vi "MODBUS  SLAVE.vi"() -> (3 "values to write":u16[](array[numeric]) caption="待写入值")   [LabVIEW 2016]
uses:
  <vilib>/Modbus/subvis/Data and Functions/Device Data Model/Device Data Model.lvclass
  <vilib>/Modbus/slave/Create Slave Instance (TCP).vi
  <vilib>/Modbus/slave/Modbus Slave.lvclass
  API/CodCr/CodCr.lvlib
panel:
  out "运行周期":u16[](array[numeric])
  in  "write operation starting address":u16=100 caption="写操作起始地址"
  out "单仪器启动命令":u16[](array[numeric])
  out "系统启动命令":u16[](array[numeric])
  in  "停止":bool
  out "register values":u16[](array[numeric]) caption="寄存器值"
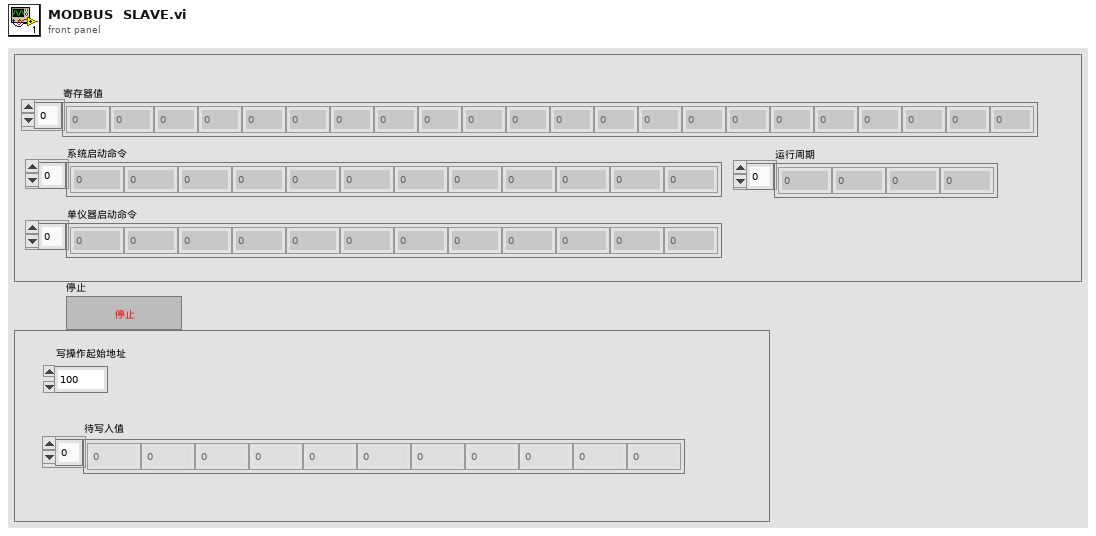
[diagram p1: front panel]
types:
  T1 = cluster{"测量模式":enum16{"水样测量", "标样核查", "零点核查", "跨度核查", "空白测试", "加标回收", "平行样", "校零", "校标"}}
  T2 = cluster{"站号":u16, "量程切换":enum32{"H", "L", "AUTO"}, "控制命令":enum16{"启动测量", "标样核查", "零点核查", "跨度核查", "空白测试", "平行样测试", "加标回收", "空白校准", "标样校准", "初始化（清洗）", "停止测试", "仪器重启", "校时", "模式设置", "测量间隔设置"}, "模式设置":enum16{"待机", "连续模式", "周期模式", "定点模式", "受控模式", "手动模式"}, "测量间隔":u16}
  T3 = cluster{"测量模式":enum16{"水样测量", "标样核查", "零点核查", "跨度核查", "加标回收", "平行样", "校零", "校标"}}
  T4 = cluster{"系统时间":timestamp, "工作状态":enum16{"空闲", "水样测试", "标样核查", "零点核查", "跨度核查", "空白测试", "平行样测试", "加标回收", "空白校准", "标样校准", "初始化（清洗）"}, "测量模式":enum16{"待机", "连续模式", "周期模式", "定点模式", "受控模式", "手动模式"}, "告警代码":enum16{"无告警", "缺试剂告警", "缺水样告警", "缺蒸馏水告警", "缺标液告警", "仪表漏液告警", "标定异常告警", "超量程告警", "加热异常", "低试剂预警", "超上限告警", "超下限告警", "仪表内部其他异常", "滴定异常告警", "电极异常告警", "量程切换告警", "参数设置告警", "PH电极电位异常", "电导率电极异常", "浊度光度异常", "溶解氧电极异常", "溶解氧光强异常", "温度异常告警", "PH异常告警", "溶解氧异常告警", "电导率异常告警", "浊度异常告警", "叶绿素异常告警", "藻密度异常告警", "蓝绿藻异常告警", "ORP异常告警", "氨氮异常告警", "清洁刷异常告警", "SD卡异常告警", "蓝牙异常告警", "Wifi异常告警", "流程异常告警"}, "故障代码":enum16{"无故障", "电机故障", "温度故障", "通讯故障", "滴定故障"}, "日志代码":u16, "软件版本":u16, "F0":sgl, "F1":sgl, "F2":sgl, "F3":sgl, "T":sgl, "H":sgl, "id":u16, "flowid":u16, "量程":u16, "总磷控温温度1":sgl, "营养盐控温温度2":sgl, "ADC":sgl}
  T5 = enum16{"空闲", "水样测试", "标样核查", "零点核查", "跨度核查", "空白测试", "平行样测试", "加标回收", "空白校准", "标样校准", "初始化（清洗）"}
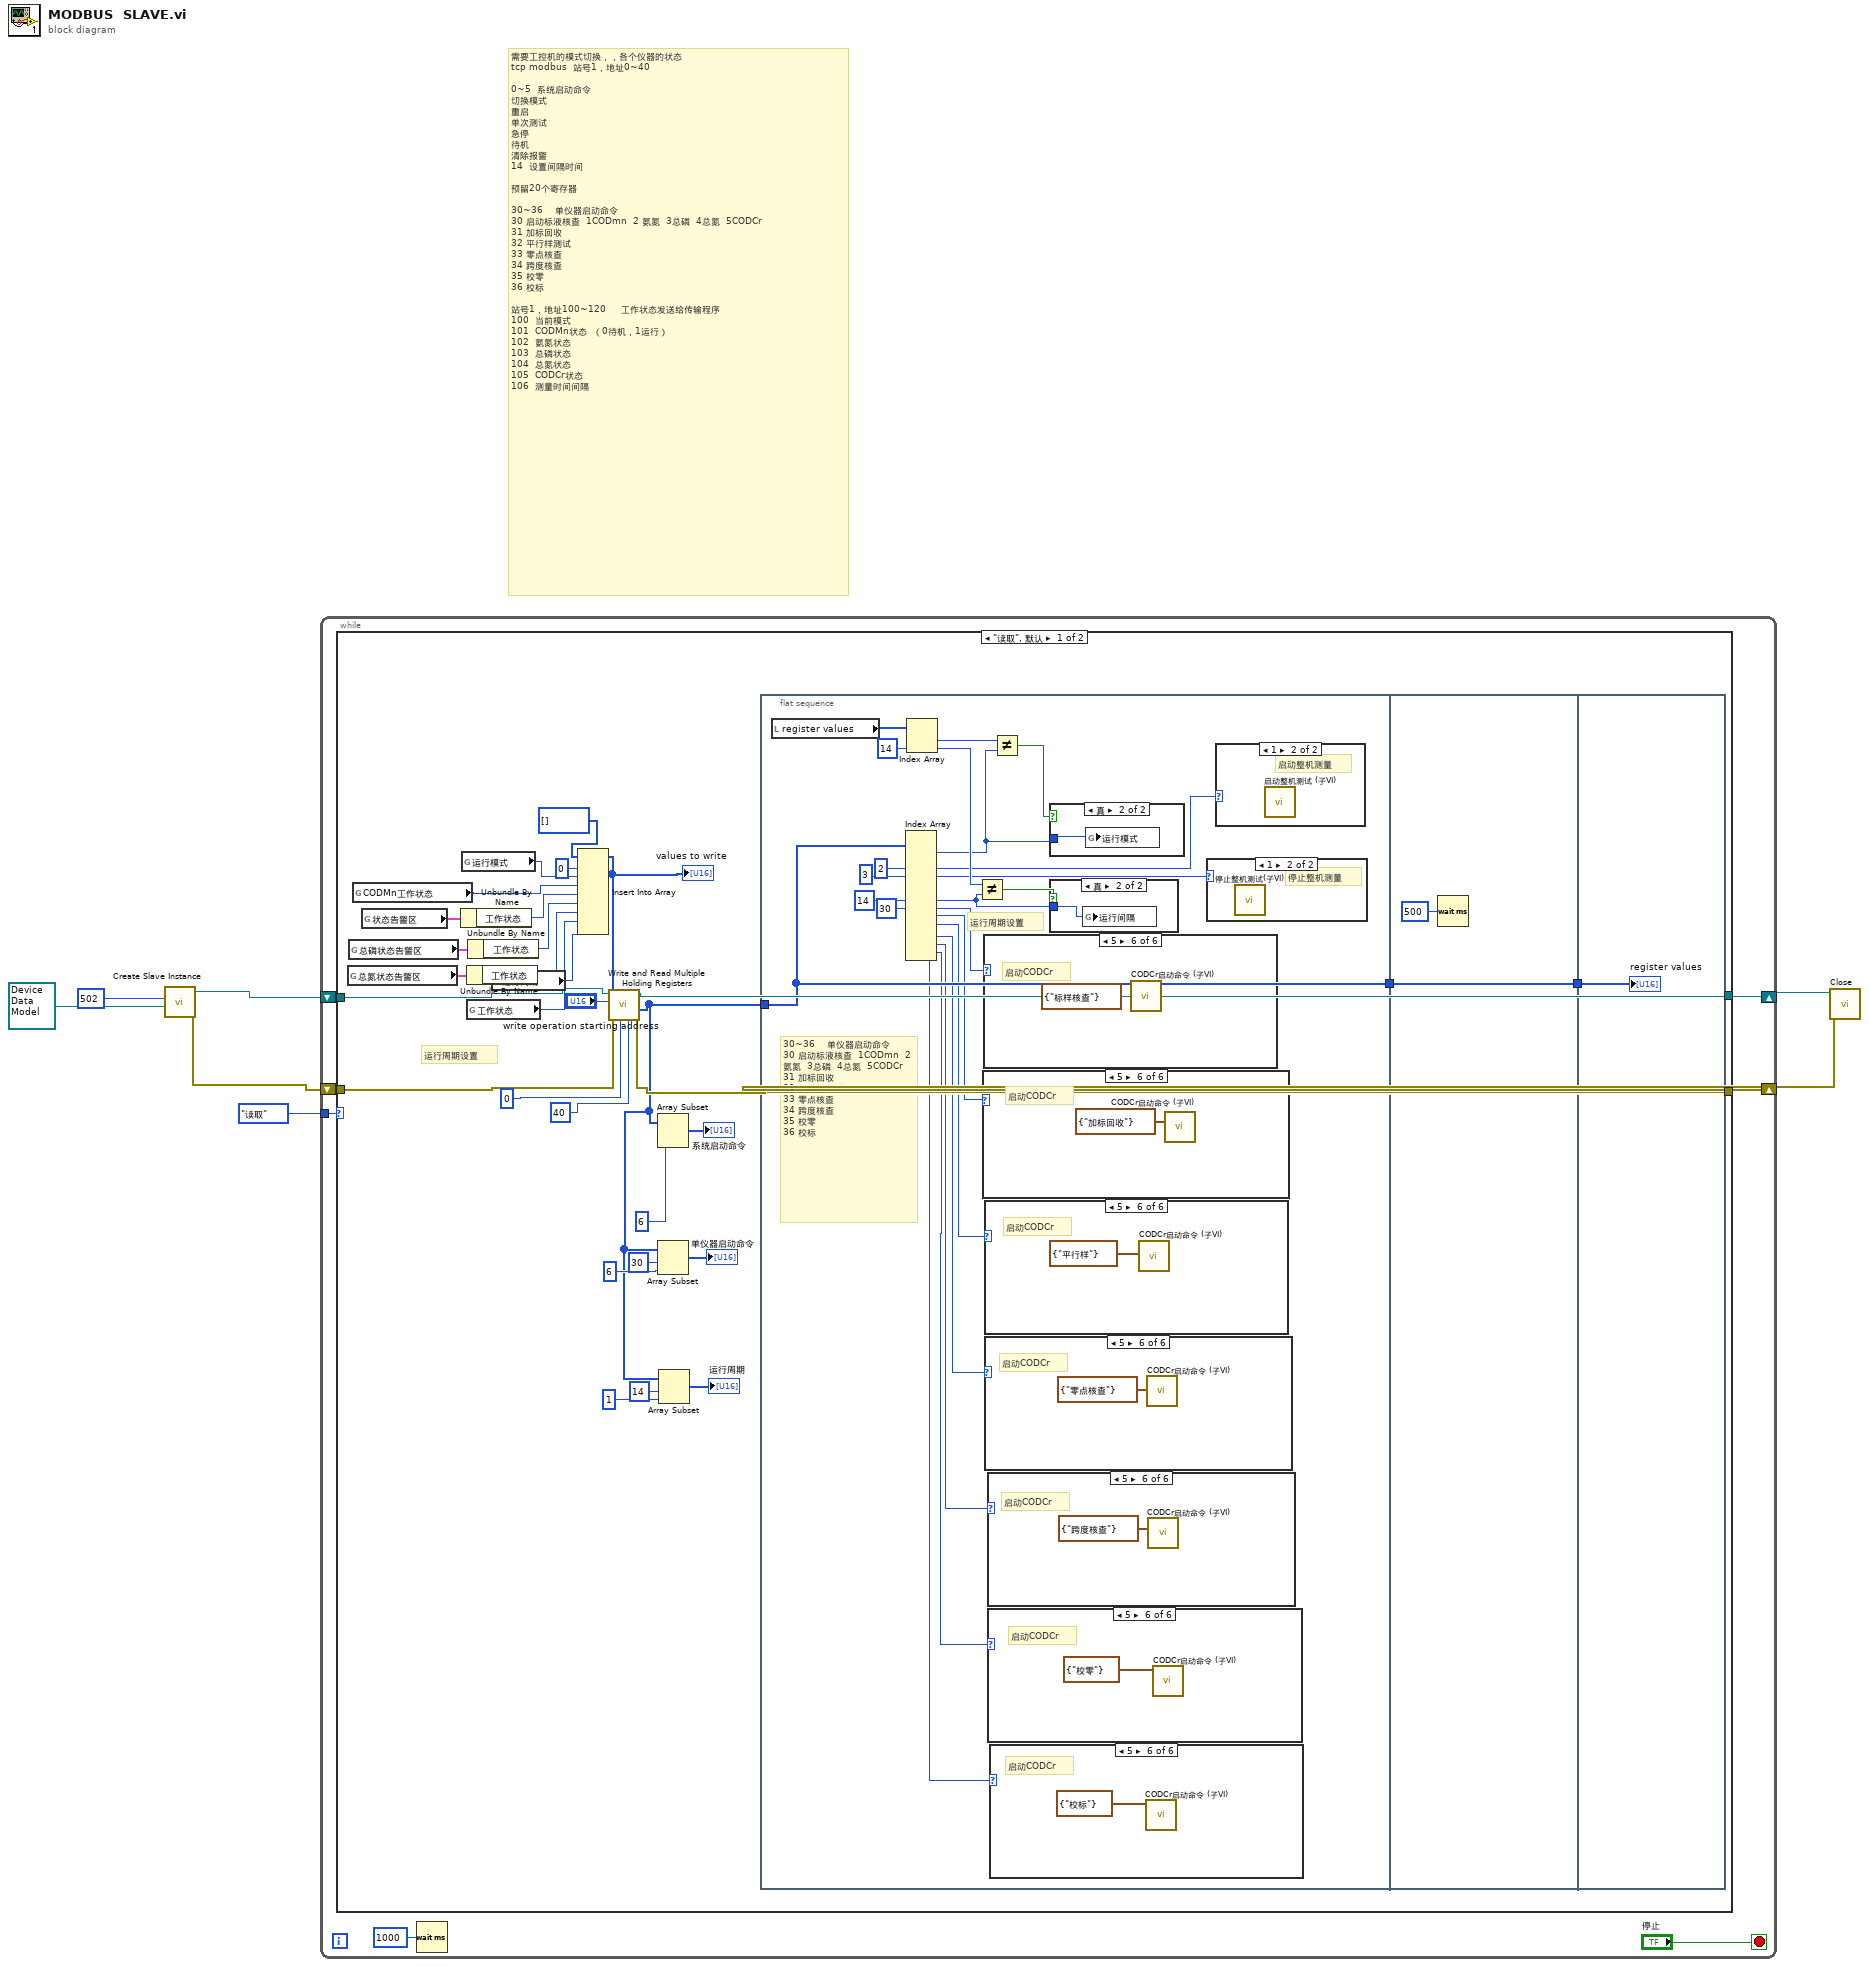
[diagram p0: block diagram]
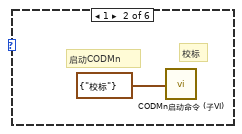
[diagram p3: hidden frame]
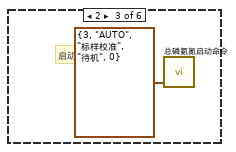
[diagram p4: hidden frame]
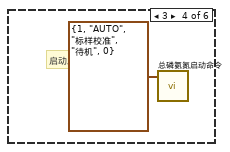
[diagram p5: hidden frame]
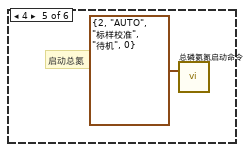
[diagram p6: hidden frame]
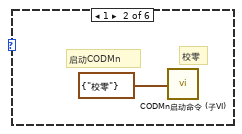
[diagram p8: hidden frame]
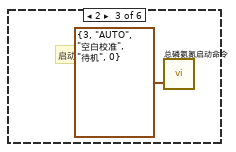
[diagram p9: hidden frame]
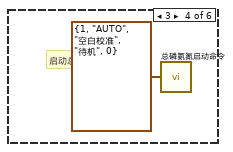
[diagram p10: hidden frame]
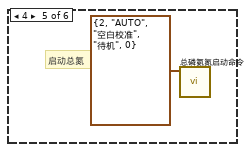
[diagram p11: hidden frame]
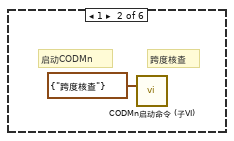
[diagram p13: hidden frame]
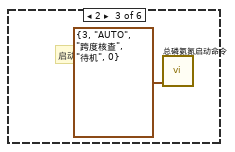
[diagram p14: hidden frame]
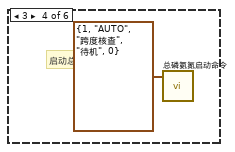
[diagram p15: hidden frame]
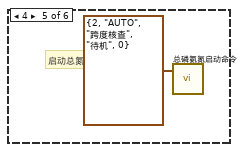
[diagram p16: hidden frame]
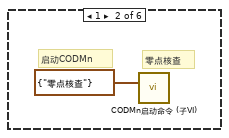
[diagram p18: hidden frame]
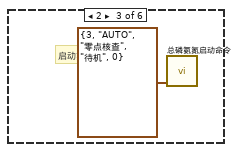
[diagram p19: hidden frame]
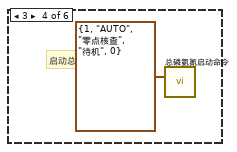
[diagram p20: hidden frame]
diagram:
  # "需要工控机的模式切换，，各个仪器的状态\ntcp modbus  站号1，地址0~40\n\n0~5  系统启动命令\n切换模式\n重启\n单次测试\n急停\n待机\n清除报警\n14  设置间隔时间\n\n预留20个寄存器\n\n30~36    单仪器启动命令\n30 启动标液核查  1CODmn  2 氨氮  3总磷  4总氮  5CODCr\n31 加标回收\n32 平行样测试\n33 零点核查\n34 跨度核查\n35 校零\n36 校标\n\n站号1，地址100~120     工作状态发送给传输程序\n100  当前模式\n101  CODMn状态  （0待机，1运行）\n102  氨氮状态\n103  总磷状态\n104  总氮状态\n105  CODCr状态\n106  测量时间间隔"
  n1 = call-poly <vilib>:"Create Slave Instance.vi"("device data model"=refnum<class "Device Data Model.lvclass"> refnum, "port (502)"=u16 502) -> ("error out"=w5:errorcluster, "TCP slave instance"=w4:refnum<class "Modbus Slave.lvclass">)  [unwired: 8 in]
  n2 = while {
    shift-right: [w12] -> w3
    shift-left: w4 -> [w14]
    shift-right: [w8] -> w2
    shift-left: w5 -> [w13]
    tunnel: enum16{"读取", "写入"}."读取" -> [w9]
    stop <- "停止" stop-if-true
    n3 = case shown="\"读取\", 默认" w9 {
      tunnel: w14 -> [w41 w109]
      tunnel: w13 -> [w40 w108]
      tunnel: [w36 w109] -> w12
      tunnel: [w37 w108] -> w8
      frame "读取", Default {
        # "运行周期设置"
        n4 = global read "VAR总磷氨氮全局变量.vi" "总氮状态告警区"() -> (w19:T4)
        n5 = global read "VAR总磷氨氮全局变量.vi" "总磷状态告警区"() -> (w21:T4)
        n6 = global read "COD测量模式全局.vi" "CODMn工作状态"() -> (w17:T5)
        n7 = global read "VAR总磷氨氮全局变量.vi" "状态告警区"() -> (w23:T4)
        n8 = Unbundle By Name(w23) -> ("工作状态"=w22:T5)
        n9 = global read "系统变量.vi" "运行模式"() -> (w33:enum16{"维护模式", "常规模式", "应急模式", "质控模式"})
        n10 = Unbundle By Name(w19) -> ("工作状态"=w18:T5)
        n11 = global read "CODcr全局变量.vi" "工作状态"() -> (w16:T5)
        n12 = Unbundle By Name(w21) -> ("工作状态"=w20:T5)
        n13 = global read "系统变量.vi" "运行间隔"() -> (w15:i16)
        n14 = Insert Into Array(array=u16[] [] ("values to write"), index=0 ("索引"), new element #1=w33, new element #2=w17, new element #3=w22, new element #4=w20, new element #5=w18, new element #6=w16, new element #7=w15) -> (w31:u16[])
        "values to write" <- w31
        n15 = call-dynamic "Write and Read Multiple Holding Registers.vi"("read count"=u16 40 ("number of holding registers"), "read operation starting address"=u16 0 ("starting address"), "error in (no error)"=w40, "values to write"=w31, "write operation starting address"="write operation starting address", "Modbus slave in"=w41) -> ("error out"=w37:errorcluster, "values read"=w26:u16[], "Modbus slave out"=w36:refnum<class "Modbus Slave.lvclass">)  [unwired: 3 in]
        n16 = Array Subset(array=w26, length=6 ("长度")) -> (→"系统启动命令":u16[])  [unwired: 1 in]
        n17 = Array Subset(array=w26, index=30 ("索引"), length=6 ("长度")) -> (→"单仪器启动命令":u16[])
        n18 = Array Subset(array=w26, index=14 ("索引"), length=1 ("长度")) -> (→"运行周期":u16[])
        n19 = flat-sequence {
          tunnel: w26 -> [w67]
          tunnel: [w67] -> w25
          tunnel: w25 -> [w105]
          tunnel: [w105] -> w24
          tunnel: w24 -> [w107]
          frame #0 {
            # "运行周期设置"
            # "30~36    单仪器启动命令\n30 启动标液核查  1CODmn  2 氨氮  3总磷  4总氮  5CODCr\n31 加标回收\n32 平行样测试\n33 零点核查\n34 跨度核查\n35 校零\n36 校标"
            n20 = local read "register values"() -> (w66:u16[])
            n21 = Index Array(array=w67, index #3=2 ("索引"), index #4=3 ("索引"), index #7=14 ("索引"), index #8=30 ("索引")) -> (element #1=w54:u16, element #3=w55:u16, element #4=w56:u16, element #7=w57:u16, element #8=w52:u16, element #9=w51:u16, element #10=w50:u16, element #11=w49:u16, element #12=w48:u16, element #13=w47:u16, element #14=w46:u16)  [unwired: 10 in, 3 out]
            n22 = Index Array(array=w66, index #2=14 ("索引")) -> (element #1=w65:u16, element #2=w62:u16)  [unwired: 1 in]
            n23 = Not Equal?(x=w62, y=w57) -> (x != y?=w61:bool)
            n24 = case shown="5" w51 {
              frame 0, Default {
              }
              frame 1 {
                # "加标回收"
                # "启动CODMn"
                n25 = call "CODMn启动命令 (子VI).vi"("启动测量模式"=T1 {"测量模式"=enum."加标回收"}) -> ()  [unwired: 11 in]
              }
              frame 2 {
                # "启动氨氮"
                n26 = call "总磷氨氮启动命令.vi"("参数"=T2 {"站号"=3, "量程切换"=enum."AUTO", "控制命令"=enum."加标回收", "模式设置"=enum."待机", "测量间隔"=0}) -> ()  [unwired: 10 in, 1 out]
              }
              frame 3 {
                # "启动总磷"
                n27 = call "总磷氨氮启动命令.vi"("参数"=T2 {"站号"=1, "量程切换"=enum."AUTO", "控制命令"=enum."加标回收", "模式设置"=enum."待机", "测量间隔"=0}) -> ()  [unwired: 10 in, 1 out]
              }
              frame 4 {
                # "启动总氮"
                n28 = call "总磷氨氮启动命令.vi"("参数"=T2 {"站号"=2, "量程切换"=enum."AUTO", "控制命令"=enum."加标回收", "模式设置"=enum."待机", "测量间隔"=0}) -> ()  [unwired: 10 in, 1 out]
              }
              frame 5 {
                # "启动CODCr"
                n29 = call "CODCr启动命令 (子VI).vi"("启动测量模式"=T3 {"测量模式"=enum."加标回收"}) -> ()  [unwired: 11 in]
              }
            }
            n30 = case shown="5" w52 {
              frame 0, Default {
              }
              frame 1 {
                # "启动标液核查"
                # "启动CODMn"
                n31 = call "CODMn启动命令 (子VI).vi"("启动测量模式"=T1 {"测量模式"=enum."标样核查"}) -> ()  [unwired: 11 in]
              }
              frame 2 {
                # "启动氨氮"
                n32 = call "总磷氨氮启动命令.vi"("参数"=T2 {"站号"=3, "量程切换"=enum."AUTO", "控制命令"=enum."标样核查", "模式设置"=enum."待机", "测量间隔"=0}) -> ()  [unwired: 10 in, 1 out]
              }
              frame 3 {
                # "启动总磷"
                n33 = call "总磷氨氮启动命令.vi"("参数"=T2 {"站号"=1, "量程切换"=enum."AUTO", "控制命令"=enum."标样核查", "模式设置"=enum."待机", "测量间隔"=0}) -> ()  [unwired: 10 in, 1 out]
              }
              frame 4 {
                # "启动总氮"
                n34 = call "总磷氨氮启动命令.vi"("参数"=T2 {"站号"=2, "量程切换"=enum."AUTO", "控制命令"=enum."标样核查", "模式设置"=enum."待机", "测量间隔"=0}) -> ()  [unwired: 10 in, 1 out]
              }
              frame 5 {
                # "启动CODCr"
                n35 = call "CODCr启动命令 (子VI).vi"("启动测量模式"=T3 {"测量模式"=enum."标样核查"}) -> ()  [unwired: 11 in]
              }
            }
            n36 = case shown="5" w50 {
              frame 0, Default {
              }
              frame 1 {
                # "平行样测试"
                # "启动CODMn"
                n37 = call "CODMn启动命令 (子VI).vi"("启动测量模式"=T1 {"测量模式"=enum."平行样"}) -> ()  [unwired: 11 in]
              }
              frame 2 {
                # "启动氨氮"
                n38 = call "总磷氨氮启动命令.vi"("参数"=T2 {"站号"=3, "量程切换"=enum."AUTO", "控制命令"=enum."平行样测试", "模式设置"=enum."待机", "测量间隔"=0}) -> ()  [unwired: 10 in, 1 out]
              }
              frame 3 {
                # "启动总磷"
                n39 = call "总磷氨氮启动命令.vi"("参数"=T2 {"站号"=1, "量程切换"=enum."AUTO", "控制命令"=enum."平行样测试", "模式设置"=enum."待机", "测量间隔"=0}) -> ()  [unwired: 10 in, 1 out]
              }
              frame 4 {
                # "启动总氮"
                n40 = call "总磷氨氮启动命令.vi"("参数"=T2 {"站号"=2, "量程切换"=enum."AUTO", "控制命令"=enum."平行样测试", "模式设置"=enum."待机", "测量间隔"=0}) -> ()  [unwired: 10 in, 1 out]
              }
              frame 5 {
                # "启动CODCr"
                n41 = call "CODCr启动命令 (子VI).vi"("启动测量模式"=T3 {"测量模式"=enum."平行样"}) -> ()  [unwired: 11 in]
              }
            }
            n42 = case shown="5" w49 {
              frame 0, Default {
              }
              frame 1 {
                # "零点核查"
                # "启动CODMn"
                n43 = call "CODMn启动命令 (子VI).vi"("启动测量模式"=T1 {"测量模式"=enum."零点核查"}) -> ()  [unwired: 11 in]
              }
              frame 2 {
                # "启动氨氮"
                n44 = call "总磷氨氮启动命令.vi"("参数"=T2 {"站号"=3, "量程切换"=enum."AUTO", "控制命令"=enum."零点核查", "模式设置"=enum."待机", "测量间隔"=0}) -> ()  [unwired: 10 in, 1 out]
              }
              frame 3 {
                # "启动总磷"
                n45 = call "总磷氨氮启动命令.vi"("参数"=T2 {"站号"=1, "量程切换"=enum."AUTO", "控制命令"=enum."零点核查", "模式设置"=enum."待机", "测量间隔"=0}) -> ()  [unwired: 10 in, 1 out]
              }
              frame 4 {
                # "启动总氮"
                n46 = call "总磷氨氮启动命令.vi"("参数"=T2 {"站号"=2, "量程切换"=enum."AUTO", "控制命令"=enum."零点核查", "模式设置"=enum."待机", "测量间隔"=0}) -> ()  [unwired: 10 in, 1 out]
              }
              frame 5 {
                # "启动CODCr"
                n47 = call "CODCr启动命令 (子VI).vi"("启动测量模式"=T3 {"测量模式"=enum."零点核查"}) -> ()  [unwired: 11 in]
              }
            }
            n48 = case shown="5" w48 {
              frame 0, Default {
              }
              frame 1 {
                # "跨度核查"
                # "启动CODMn"
                n49 = call "CODMn启动命令 (子VI).vi"("启动测量模式"=T1 {"测量模式"=enum."跨度核查"}) -> ()  [unwired: 11 in]
              }
              frame 2 {
                # "启动氨氮"
                n50 = call "总磷氨氮启动命令.vi"("参数"=T2 {"站号"=3, "量程切换"=enum."AUTO", "控制命令"=enum."跨度核查", "模式设置"=enum."待机", "测量间隔"=0}) -> ()  [unwired: 10 in, 1 out]
              }
              frame 3 {
                # "启动总磷"
                n51 = call "总磷氨氮启动命令.vi"("参数"=T2 {"站号"=1, "量程切换"=enum."AUTO", "控制命令"=enum."跨度核查", "模式设置"=enum."待机", "测量间隔"=0}) -> ()  [unwired: 10 in, 1 out]
              }
              frame 4 {
                # "启动总氮"
                n52 = call "总磷氨氮启动命令.vi"("参数"=T2 {"站号"=2, "量程切换"=enum."AUTO", "控制命令"=enum."跨度核查", "模式设置"=enum."待机", "测量间隔"=0}) -> ()  [unwired: 10 in, 1 out]
              }
              frame 5 {
                # "启动CODCr"
                n53 = call "CODCr启动命令 (子VI).vi"("启动测量模式"=T3 {"测量模式"=enum."跨度核查"}) -> ()  [unwired: 11 in]
              }
            }
            n54 = case shown="5" w47 {
              frame 0, Default {
              }
              frame 1 {
                # "校零"
                # "启动CODMn"
                n55 = call "CODMn启动命令 (子VI).vi"("启动测量模式"=T1 {"测量模式"=enum."校零"}) -> ()  [unwired: 11 in]
              }
              frame 2 {
                # "启动氨氮"
                n56 = call "总磷氨氮启动命令.vi"("参数"=T2 {"站号"=3, "量程切换"=enum."AUTO", "控制命令"=enum."空白校准", "模式设置"=enum."待机", "测量间隔"=0}) -> ()  [unwired: 10 in, 1 out]
              }
              frame 3 {
                # "启动总磷"
                n57 = call "总磷氨氮启动命令.vi"("参数"=T2 {"站号"=1, "量程切换"=enum."AUTO", "控制命令"=enum."空白校准", "模式设置"=enum."待机", "测量间隔"=0}) -> ()  [unwired: 10 in, 1 out]
              }
              frame 4 {
                # "启动总氮"
                n58 = call "总磷氨氮启动命令.vi"("参数"=T2 {"站号"=2, "量程切换"=enum."AUTO", "控制命令"=enum."空白校准", "模式设置"=enum."待机", "测量间隔"=0}) -> ()  [unwired: 10 in, 1 out]
              }
              frame 5 {
                # "启动CODCr"
                n59 = call "CODCr启动命令 (子VI).vi"("启动测量模式"=T3 {"测量模式"=enum."校零"}) -> ()  [unwired: 11 in]
              }
            }
            n60 = case shown="5" w46 {
              frame 0, Default {
              }
              frame 1 {
                # "校标"
                # "启动CODMn"
                n61 = call "CODMn启动命令 (子VI).vi"("启动测量模式"=T1 {"测量模式"=enum."校标"}) -> ()  [unwired: 11 in]
              }
              frame 2 {
                # "启动氨氮"
                n62 = call "总磷氨氮启动命令.vi"("参数"=T2 {"站号"=3, "量程切换"=enum."AUTO", "控制命令"=enum."标样校准", "模式设置"=enum."待机", "测量间隔"=0}) -> ()  [unwired: 10 in, 1 out]
              }
              frame 3 {
                # "启动总磷"
                n63 = call "总磷氨氮启动命令.vi"("参数"=T2 {"站号"=1, "量程切换"=enum."AUTO", "控制命令"=enum."标样校准", "模式设置"=enum."待机", "测量间隔"=0}) -> ()  [unwired: 10 in, 1 out]
              }
              frame 4 {
                # "启动总氮"
                n64 = call "总磷氨氮启动命令.vi"("参数"=T2 {"站号"=2, "量程切换"=enum."AUTO", "控制命令"=enum."标样校准", "模式设置"=enum."待机", "测量间隔"=0}) -> ()  [unwired: 10 in, 1 out]
              }
              frame 5 {
                # "启动CODCr"
                n65 = call "CODCr启动命令 (子VI).vi"("启动测量模式"=T3 {"测量模式"=enum."校标"}) -> ()  [unwired: 11 in]
              }
            }
            n66 = Not Equal?(x=w65, y=w54) -> (x != y?=w64:bool)
            n67 = case shown="真" w64 {
              tunnel: w54 -> [_ w104]
              frame False {
              }
              frame True {
                n68 = global write "系统变量.vi" "运行模式"(w104) -> ()
              }
            }
            n69 = case shown="真" w61 {
              tunnel: w57 -> [_ w103]
              frame False {
              }
              frame True {
                n70 = global write "系统变量.vi" "运行间隔"(w103) -> ()
              }
            }
            n71 = case shown="1" w56 {
              frame 0, Default {
              }
              frame 1 {
                # "停止整机测量"
                n72 = call "停止整机测试(子VI).vi"() -> ()  [unwired: 12 in]
              }
            }
            n73 = case shown="1" w55 {
              frame 0, Default {
              }
              frame 1 {
                # "启动整机测量"
                n74 = call "启动整机测试 (子VI).vi"() -> ()  [unwired: 12 in]
              }
            }
          }
          frame #1 {
            n75 = Wait (ms)(milliseconds to wait=u32 500 ("等待时间（毫秒）")) -> ()  [unwired: 1 out]
          }
          frame #2 {
            "register values" <- w107
          }
        }
      }
      frame "写入" {
      }
    }
    n76 = Wait (ms)(milliseconds to wait=u32 1000 ("等待时间（毫秒）")) -> ()  [unwired: 1 out]
  }
  n77 = call-dynamic "Close.vi"("error in (no error)"=w2, "Modbus slave in"=w3) -> ()  [unwired: 9 in, 1 out]
